vi "Test Probe on Wire Exists - no probes.vi"() -> (0 "error out":errorcluster)   [LabVIEW 2020]
doc: "Test of <b>Probe on Wire Exists.vi</b>: check the VI detects no probes."
uses:
  <vilib>/Utility/traverseref.llb/TRef TravTarget.ctl
  src/Type Definitions/Class Name--enum.ctl
  <vilib>/addons/_JKI Toolkits/Caraya/classes/Assert/Assert False.vi
  <vilib>/addons/_JKI Toolkits/Caraya/classes/Test/Test.lvclass
  <vilib>/addons/_JKI Toolkits/Caraya/classes/Assert/Assert.lvclass
  <vilib>/Utility/traverseref.llb/VI Scripting - Traverse.lvlib
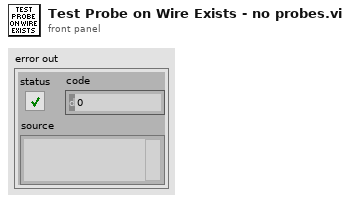
[diagram p1: front panel]
types:
  T1 = typedef "Class Name--enum.ctl" = enum16{"Node", "Wire"}
  T2 = typedef "TRef TravTarget.ctl" = enum16{"FP", "BD", "Other"}
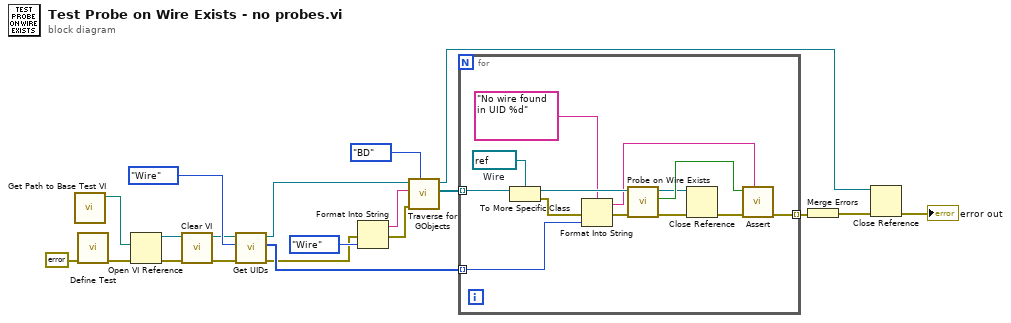
[diagram p0: block diagram]
diagram:
  n1 = call "Get Path to Base Test VI.vi"() -> ("Path"=w19:path)  [unwired: 11 in]
  n2 = call <vilib>:"Define Test.vi"("error in (no error)"=errorcluster {"status"=FALSE, "code"=0, "source"=""}) -> ("error out"=w5:errorcluster)  [unwired: 9 in, 1 out]
  n3 = Open VI Reference(vi path=w19, error in (no error)=w5) -> (vi reference=w4:refnum<vi>, error out=w2:errorcluster)  [unwired: 4 in]
  n4 = call "Clear VI.vi"("error in"=w2, "VI Refnum In"=w4) -> ("error out"=w1:errorcluster, "VI Refnum Out"=w3:refnum<vi>)  [unwired: 8 in]
  n5 = call "Get UIDs.vi"("error in"=w1, "Class Name"=Class_Name--enum."Wire", "VI Refnum In"=w3) -> ("error out"=w7:errorcluster, "UIDs"=w9:i32[], "VI Refnum Out"=w6:refnum<vi>)  [unwired: 6 in]
  n6 = Format Into String(error in=w7, Class_Name--enum."Wire" ("Class Name")) -> (resulting string=w16:string, error out=w15:errorcluster)  [unwired: 2 in]
  n7 = call <vilib>:"Traverse for GObjects.vi"("Traverse Target"=TRef_TravTarget."BD", "error in (no error)"=w15, "Class Name"=w16, "VI Refnum"=w6) -> ("References"=w14:refnum<vi>[], "dup VI Refnum"=w10:refnum<vi>)  [unwired: 4 in, 2 out]
  n8 = for {
    tunnel: w14 -> [w33] mode=indexing
    tunnel: w9 -> [w28] mode=indexing
    tunnel: [w24] -> w13 mode=indexing
    w32 = refnum<vi> refnum  # Wire
    n9 = To More Specific Class(target class=w32, reference=w33) -> (specific class reference=w31:refnum<vi>, error out=w27:errorcluster)  [unwired: 1 in]
    n10 = Format Into String(format string="No wire found in UID %d", error in=w27, w28) -> (resulting string=w25:string, error out=w26:errorcluster)  [unwired: 1 in]
    n11 = call "Probe on Wire Exists.vi"("error in"=w26, "Wire in"=w31) -> ("error out"=w22:errorcluster, "Probe Exists"=w30:bool, "Wire out"=w23:refnum<vi>)  [unwired: 6 in, 1 out]
    n12 = Close Reference(reference=w23, error in (no error)=w22) -> (error out=w21:errorcluster)
    n13 = call-poly <vilib>:"Assert.vi"("Label"=w25, "error in (no error)"=w21, "False?"=w30) -> ("error out"=w24:errorcluster)  [unwired: 7 in, 1 out]
  }
  n14 = Merge Errors(w13) -> (w12:errorcluster)
  n15 = Close Reference(reference=w10, error in (no error)=w12) -> (error out=→"error out":errorcluster)
